vi "LoopState.vi"(8 "error in (no error)":errorcluster, 9 "loop action":string, 10 "process name":string, 11 "Qbus in":refnum<class "Qbus.lvclass">) -> (0 "error out":errorcluster, 3 "Qbus out":refnum<class "Qbus.lvclass">)   [LabVIEW 2017, in "TraceLogger.lvlib"]
uses:
  <vilib>/addons/TraceLogger/TraceLogger.lvlib
  <vilib>/addons/Qbus/Qbus.lvclass
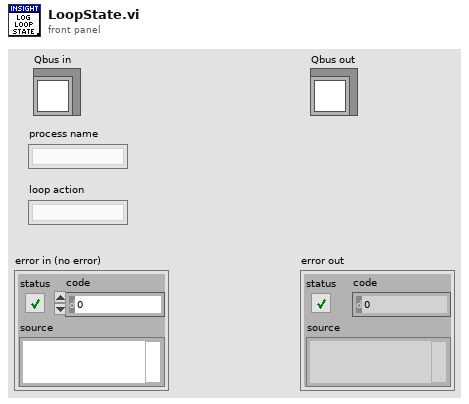
[diagram p1: front panel]
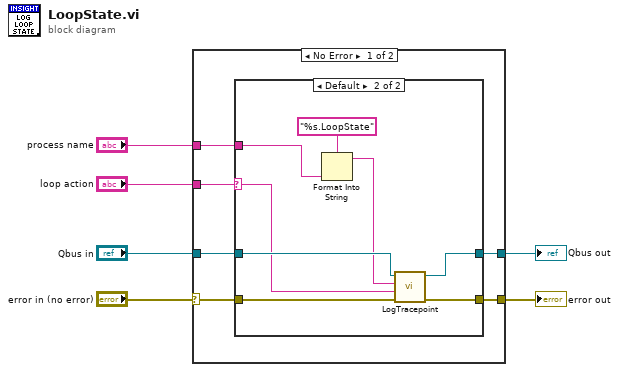
[diagram p0: block diagram]
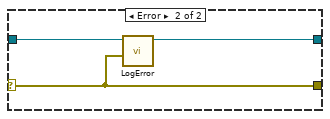
[diagram p3: hidden frame]
diagram:
  n1 = case shown="No Error" "error in (no error)" {
    selector: "error in (no error)" -> [w9 w23]
    tunnel: "process name" -> [w12 _]
    tunnel: "Qbus in" -> [w11 w25]
    tunnel: [w10 w24] -> w3
    tunnel: [w8 w23] -> w2
    tunnel: "loop action" -> [w7 _]
    frame No Error {
      n2 = case shown="Default" w7 {
        selector: w7 -> [_ w15]
        tunnel: w12 -> [_ w21]
        tunnel: w11 -> [w14 w20]
        tunnel: [w14 w19] -> w10
        tunnel: w9 -> [w13 w18]
        tunnel: [w13 w17] -> w8
        frame "" {
        }
        frame Default {
          n3 = Format Into String(format string="%s.LoopState", w21) -> (resulting string=w16:string)  [unwired: 2 in, 1 out]
          n4 = call <vilib>:"LogTracepoint.vi"("error in (no error)"=w18, "log string"=w15, "tracepoint"=w16, "qbus in"=w20) -> ("error out"=w17:errorcluster, "qbus out"=w19:refnum<class "Qbus.lvclass">)  [unwired: 6 in]
        }
      }
    }
    frame Error {
      n5 = call <vilib>:"LogError.vi"("error"=w23, "qbus in"=w25) -> ("qbus out"=w24:refnum<class "Qbus.lvclass">)  [unwired: 8 in, 1 out]
    }
  }
  "error out" <- w2
  "Qbus out" <- w3
